vi "SPD.HV_Grid Check HV_bias Limits.vi"(8 "Error In":errorcluster, 10 "HV_GridParams":T1, 11 "Next HV_bias":dbl) -> (0 "Error Out":errorcluster)   [LabVIEW 2018]
uses:
  typedefs/SPD.HV_Grid Test Params.ctl
  <vilib>/Utility/error.llb/Error Cluster From Error Code.vi
  <vilib>/ErrorRing/Error Ring.xnode
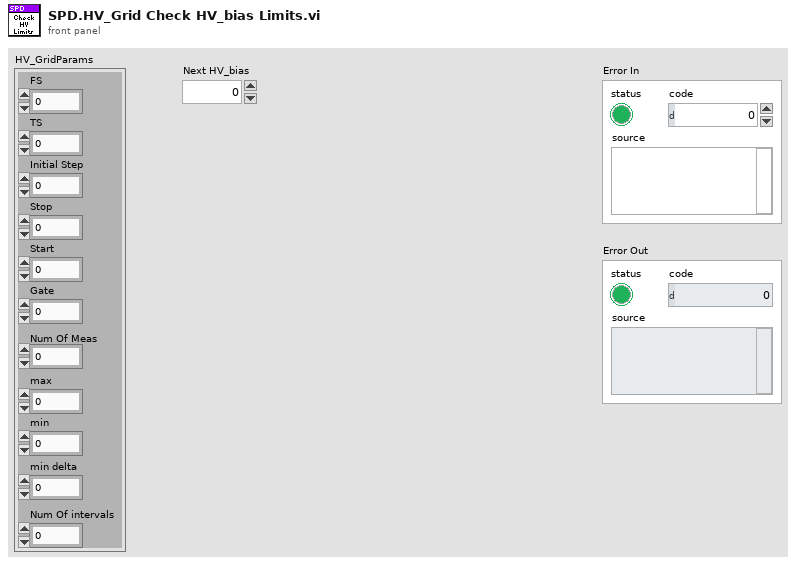
[diagram p1: front panel]
types:
  T1 = typedef "SPD.HV_Grid Test Params.ctl" = cluster{"FS":i32, "TS":i32, "Initial Step":dbl, "Stop":dbl, "Start":dbl, "Gate":dbl, "Num Of Meas":i32, "max":dbl, "min":dbl, "min delta":dbl, "Num Of intervals":i32}
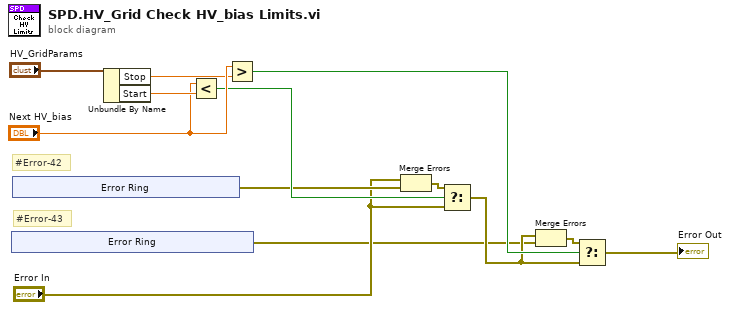
[diagram p0: block diagram]
diagram:
  # "#Error-43"
  # "#Error-42"
  n1 = xnode "Error Ring"() -> ("error out"=w2:errorcluster)
  n2 = xnode "Error Ring"() -> ("error out"=w8:errorcluster)
  n3 = Unbundle By Name("HV_GridParams") -> ("Stop"=w10:dbl, "Start"=w12:dbl)
  n4 = Less?(x="Next HV_bias", y=w12) -> (x < y?=w9:bool)
  n5 = Greater?(x="Next HV_bias", y=w10) -> (0:w4:bool)
  n6 = Merge Errors("Error In", w8) -> (w7:errorcluster)
  n7 = Select(t=w7, s=w9, f="Error In") -> (s? t:f=w3:errorcluster)
  n8 = Merge Errors(w3, w2) -> (w5:errorcluster)
  n9 = Select(t=w5, s=w4, f=w3) -> (s? t:f=→"Error Out":errorcluster)
